vi "Read Raw Data.vi"(8 "error in (no error)":errorcluster, 10 "Previous Partial Sentence":string, 11 "VISA resource name":refnum<visa-resource-name>) -> (0 "error out":errorcluster, 1 "Complete NMEA Sentences":string[](array[string]), 2 "Remaining Partial Sentence":string, 3 "VISA resource name out":refnum<visa-resource-name>)   [LabVIEW 2009]
doc: "Reads raw sentences from the u-blox device. Use this VI if data is required that is not included in or more specific than the outputs of Read GPS Data.vi. See u-blox 5 Series Acquire and Chart GPS Advanced.vi for an example of how to use this VI."
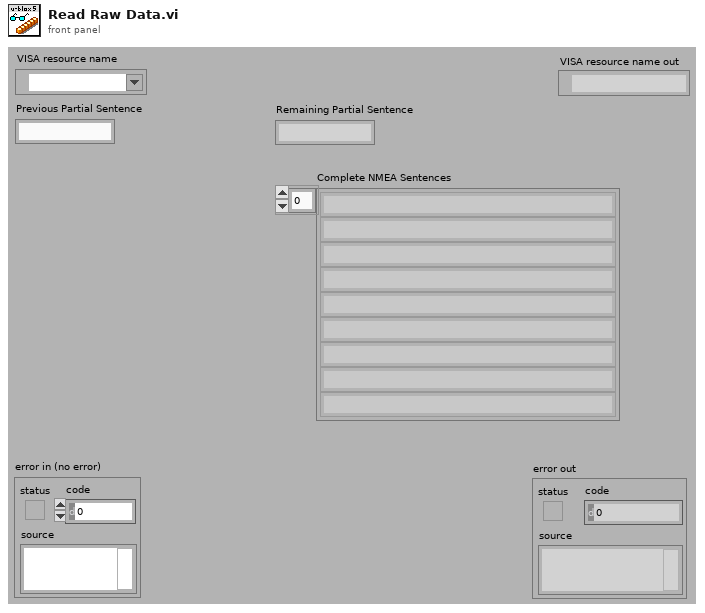
[diagram p1: front panel]
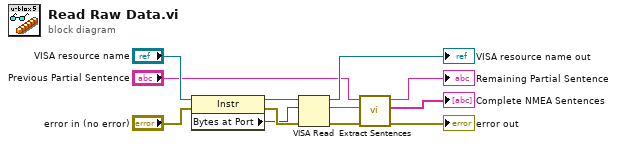
[diagram p0: block diagram]
diagram:
  n1 = property class="Instr"(reference="VISA resource name", error in="error in (no error)") -> (reference out=w8:refnum<visa-resource-name>, error out=w10:errorcluster, "Bytes at Port"=w7:u32)
  n2 = VISA Read(VISA resource name=w8, byte count=w7, error in (no error)=w10) -> (VISA resource name out=→"VISA resource name out":refnum<visa-resource-name>, read buffer=w2:string, error out=w3:errorcluster)  [unwired: 1 out]
  n3 = call "Extract Sentences.vi"("error in (no error)"=w3, "sensor data"=w2, "previous partial sentence"="Previous Partial Sentence") -> ("error out"=→"error out":errorcluster, "complete sentences"=→"Complete NMEA Sentences":string[], "remaining partial sentence"=→"Remaining Partial Sentence":string)  [unwired: 4 in, 2 out]
